vi "StraightDrive.vi"(9 "RightDrive in":dbl, 10 "LeftDrive in":dbl, 11 "StraightDrive":bool) -> (1 "RightDrive out":dbl, 2 "LeftDrive out":dbl)   [LabVIEW 2015]
doc: "When StraightDrive is true, takes the joystick that is greater (in absolute value) and sets both joysticks to that value."
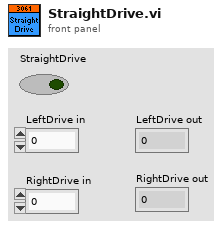
[diagram p1: front panel]
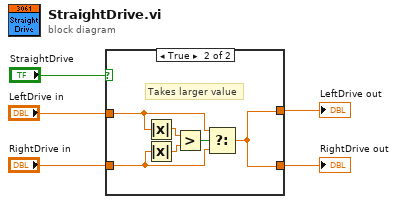
[diagram p0: block diagram]
diagram:
  n1 = case shown="True" "StraightDrive" {
    tunnel: [w7 w13] -> w4
    tunnel: "RightDrive in" -> [w7 w9]
    tunnel: [w6 w13] -> w5
    tunnel: "LeftDrive in" -> [w6 w10]
    frame False {
    }
    frame True {
      # "Takes larger value"
      n2 = Absolute Value(x=w10) -> (abs(x)=w11:dbl)
      n3 = Absolute Value(x=w9) -> (abs(x)=w8:dbl)
      n4 = Greater?(x=w11, y=w8) -> (0:w12:bool)
      n5 = Select(t=w10, s=w12, f=w9) -> (s? t:f=w13:dbl)
    }
  }
  "LeftDrive out" <- w5
  "RightDrive out" <- w4
